vi "Get VS Amplitude Value.vi"(10 "value":i32, 11 "index":i32) -> (2 "value out":i32, 3 "function return":u32)   [LabVIEW 2018, in "Copy of Andor SDK.lvlib"]
doc: "EXPNETTYPE unsigned int WINAPI GetVSAmplitudeValue(int index, int * value);"
uses:
  Copy of Andor SDK.lvlib
  <userlib>/Andor SDK/ATMCD32D.dll
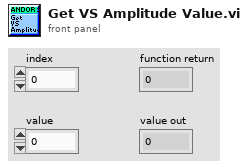
[diagram p1: front panel]
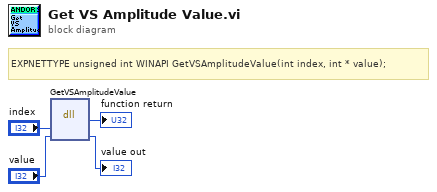
[diagram p0: block diagram]
diagram:
  # "EXPNETTYPE unsigned int WINAPI GetVSAmplitudeValue(int index, int * value);"
  n1 = dll-call lib="C:/Program Files (x86)/National Instruments/LabVIEW 2018/user.lib/Andor SDK/ATMCD32D.*" fn="GetVSAmplitudeValue"("index"="index", "value"="value") -> (→"function return":u32, "value"=→"value out":i32)  [unwired: 4 in, 2 out]
